vi "WriteDictionary.vi"(8 "error in (no error)":errorcluster, 10 "Localization":T1, 11 "Dictionary Path":path) -> (0 "error out":errorcluster, 2 "CSV String":string, 3 "Dictionary Path Dup":path)   [LabVIEW 2019]
uses:
  Dictionary--Cluster.ctl
  Font -- Cluster.ctl
  Phrase Dictionary Entry -- Cluster.ctl
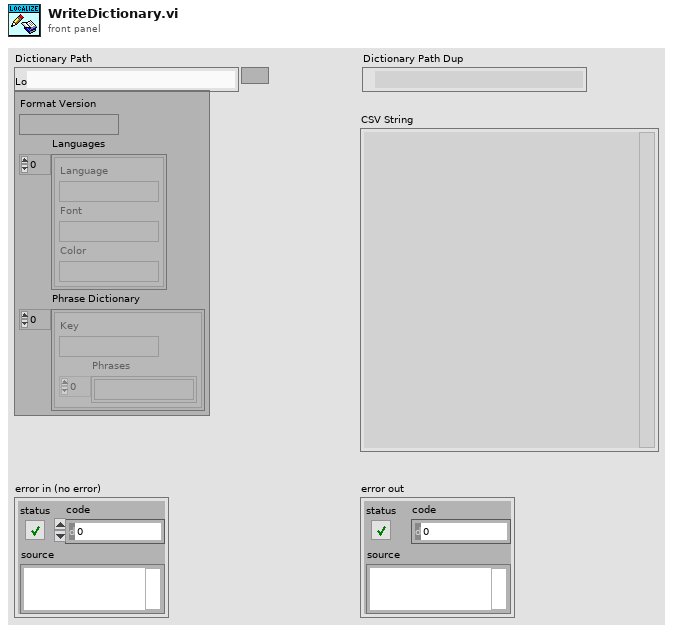
[diagram p1: front panel]
types:
  T1 = typedef "Dictionary--Cluster.ctl" = cluster{"Format Version":string, "Languages":T2[], "Phrase Dictionary":T3[]}
  T2 = typedef "Font -- Cluster.ctl" = cluster{"Language":string, "Font":string, "Color":string}
  T3 = typedef "Phrase Dictionary Entry -- Cluster.ctl" = cluster{"Key":string, "Phrases":string[]}
  T4 = enum16{"open", "replace", "create", "open or create", "replace or create", "replace or create with confirmation"}
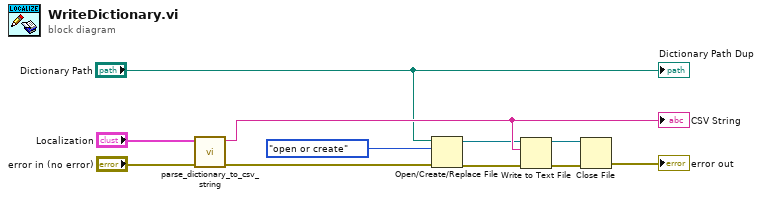
[diagram p0: block diagram]
diagram:
  n1 = call "parse_dictionary_to_csv_string.vi"("error in (no error)"="error in (no error)", "Localization"="Localization") -> ("error out"=w7:errorcluster, "CSV String"=w8:string)  [unwired: 8 in]
  "CSV String" <- w8
  n2 = Open/Create/Replace File(file path (use dialog)="Dictionary Path", error in=w7, operation (0:open)=T4."open or create") -> (refnum out=w2:refnum<file>, error out=w1:errorcluster)  [unwired: 3 in, 1 out]
  n3 = Write to Text File(file (use dialog)=w2, text=w8, error in=w1) -> (refnum out=w3:refnum<file>, error out=w4:errorcluster)  [unwired: 1 in, 1 out]
  n4 = Close File(refnum=w3, error in=w4) -> (error out=→"error out":errorcluster)  [unwired: 1 out]
  "Dictionary Path Dup" <- "Dictionary Path"
